vi "Control Auto Shooter.vi"(11 "Avoid Race Condition":bool) -> ()   [LabVIEW 2020]
uses:
  Framework/Robot Global Data.vi
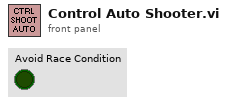
[diagram p1: front panel]
types:
  T1 = typedef "Command Status Info.ctl" = cluster{"Name":string, "Status":T2, "notifier out":T3}
  T2 = typedef "Completion Status.ctl" = enum16{"Successful", "Aborted", "Incomplete"}
  T3 = typedef "Completion Notifier.ctl" = refnum<notifier>
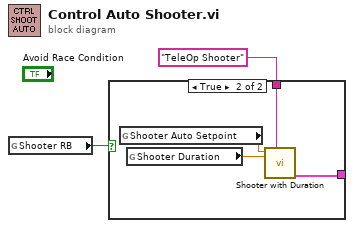
[diagram p0: block diagram]
diagram:
  n1 = global read "Robot Global Data.vi" "Shooter RB"() -> (w1:bool)
  n2 = case shown="True" w1 {
    tunnel: "TeleOp Shooter" ("Description") -> [_ w4]
    tunnel: [_ w3] -> _
    frame False {
    }
    frame True {
      n3 = global read "Robot Global Data.vi" "Shooter Auto Setpoint"() -> (w5:dbl)
      n4 = global read "Robot Global Data.vi" "Shooter Duration"() -> (w6:dbl)
      n5 = call "Shooter with Duration .vi"("Description"=w4, "Duration (s)"=w6, "Setpoint"=w5) -> ("Command Info Out"=w3:T1)  [unwired: 8 in]
    }
  }
